vi "Daten Serialisieren - 2xU32.vi"(9 "Frame-ID":u32[](array[numeric]), 10 "Aktuelle Zeit":timestamp, 11 "Messdaten":sgl[](array[numeric])) -> (2 "data":T1[](array[typedef])=[{"timestamp"=timestamp(0 s since 1904-01-01), "payload"=[0, 2, 3, 4, 5, 6, 7, 8], "identifier"=2, "type"=0, "extended?"=FALSE, "echo?"=FALSE}, {"timestamp"=timestamp(0 s since 1904-01-01), "payload"=[0, 1, 2, 3, 4, 5, 6, 7], "identifier"=3, "type"=0, "extended?"=FALSE, "echo?"=FALSE}] {"payload" format="%x"; "timestamp" format="%<%.7X\n%x>T"; "type" items=["CAN Data"=0, "CAN Remote"=1, "CAN Bus Error"=2, "CAN 2.0 Data"=8, "CAN FD Data"=16, "CAN FD+BRS Data"=24, "J1939 Data"=192, "Delay"=224, "Log Trigger"=225, "Start Trigger"=226]; "identifier" format="%x"})   [LabVIEW 2020, in "CAN Interface.lvlib"]
uses:
  CAN Interface.lvlib
  <vilib>/xnet/xnet.llb/XNET Frame CAN.ctl
  <vilib>/xnet/xnet.llb/XNET Frame Type CAN.ctl
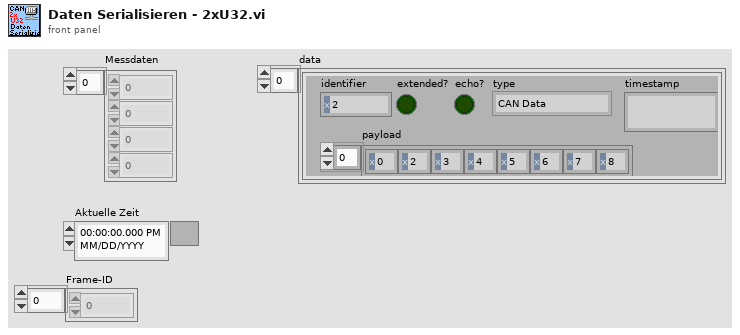
[diagram p1: front panel]
types:
  T1 = typedef "XNET Frame CAN.ctl" = cluster{"timestamp":timestamp, "payload":u8[], "identifier":u32, "type":T2, "extended?":bool, "echo?":bool}
  T2 = typedef "XNET Frame Type CAN.ctl" = u8
  T3 = enum16{"big-endian, network order", "native, host order", "little-endian"}
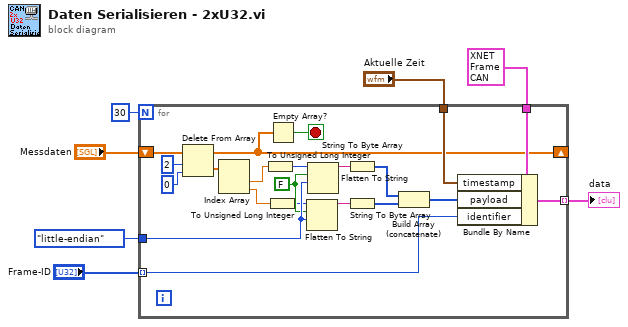
[diagram p0: block diagram]
diagram:
  n1 = for {
    N: 30 -> [_]
    tunnel: T3."little-endian" ("Byte-Reihenfolge (0:Big-Endian, Netzwerkreihenfolge)") -> [w14]
    tunnel: T1 {"timestamp"=timestamp(0 s since 1904-01-01), "payload"=[0, 2, 3, 4, 5, 6, 7, 8], "identifier"=2, "type"=0, "extended?"=FALSE, "echo?"=FALSE} ("CAN frame") -> [w27]
    tunnel: "Frame-ID" -> [w8] mode=indexing
    tunnel: "Aktuelle Zeit" -> [w26]
    tunnel: [w25] -> w3 mode=indexing
    shift-right: [w16] -> _
    shift-left: "Messdaten" -> [w24]
    stop <- w15 stop-if-true
    w13 = FALSE ("Array- oder String-Größe voranstellen? (T)")
    n2 = Delete From Array(array=w24, length=2 ("Länge"), index=0 ("Index")) -> (deleted portion=w21:sgl[], array with subset deleted=w16:sgl[])
    n3 = Index Array(array=w21) -> (element #1=w12:sgl, element #2=w11:sgl)  [unwired: 2 in]
    n4 = To Unsigned Long Integer(number=w12) -> (unsigned 32bit integer=w10:u32)
    n5 = To Unsigned Long Integer(number=w11) -> (unsigned 32bit integer=w9:u32)
    n6 = Empty Array?(array=w16) -> (empty?=w15:bool)
    n7 = Flatten To String(anything=w9, prepend array or string size? (T)=w13, byte order (0:big-endian, network order)=w14) -> (data string=w28:string)  [unwired: 1 in, 2 out]
    n8 = Flatten To String(anything=w10, prepend array or string size? (T)=w13, byte order (0:big-endian, network order)=w14) -> (data string=w20:string)  [unwired: 1 in, 2 out]
    n9 = String To Byte Array(string=w20) -> (unsigned byte array=w19:u8[])
    n10 = String To Byte Array(string=w28) -> (unsigned byte array=w18:u8[])
    n11 = Build Array (concatenate)(w19, w18) -> (w17:u8[])
    n12 = Bundle By Name(cluster=w27, "timestamp"=w26, "payload"=w17, "identifier"=w8) -> (w25:T1)
  }
  "data" <- w3
